vi "Init Condition.vi"(5 "Sequencing":refnum<class "MessageQ.lvclass">, 6 "Variables":refnum<class "Variables.lvclass">, 7 "VolatusAPI":refnum<class "VolatusAPI.lvclass">, 8 "error in (no error)":refnum<class "MultiErrors.lvclass">, 10 "Condition Config":refnum<class "Condition Config.lvclass">, 11 "SeqRunning Condition in":refnum<class "SeqRunning Condition.lvclass">) -> (0 "error out":refnum<class "MultiErrors.lvclass">, 3 "SeqRunning Condition out":refnum<class "SeqRunning Condition.lvclass">)   [LabVIEW 2020, in "VolatusSeq.lvlib" / "SeqRunning Condition.lvclass"]
uses:
  SeqRunning Condition.lvclass
  VolatusErrorUtilities/MultiErrors/MultiErrors.lvclass
  Volatus/VolatusAPI/VolatusAPI.lvclass
  VolatusSeqConfig/Condition Config/Condition Config.lvclass
  Volatus/MessageQ/MessageQ.lvclass
  VolatusSeqConfig/SeqRunning Condition Config/SeqRunning Condition Config.lvclass
  SeqRunning Condition.lvclass/SeqRunning Condition.ctl
  Variables/Variables.lvclass
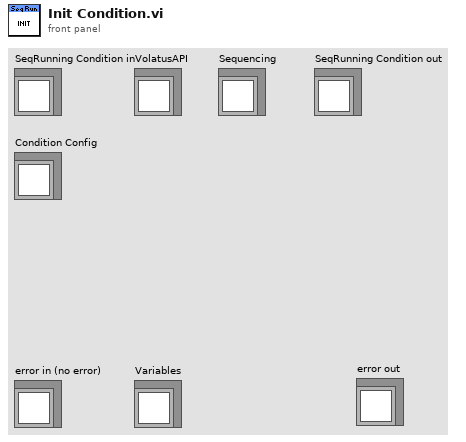
[diagram p1: front panel]
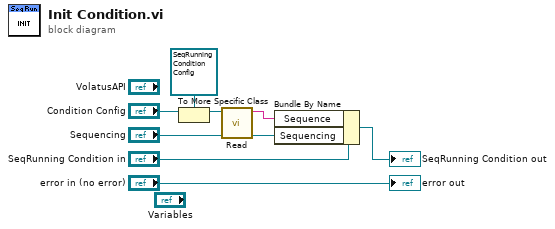
[diagram p0: block diagram]
diagram:
  n1 = To More Specific Class(target class=refnum<class "SeqRunning Condition Config.lvclass"> refnum ("VolatusSeqConfig.lvlib:SeqRunning Condition Config.lvclass"), reference="Condition Config") -> (specific class reference=w5:refnum<class "SeqRunning Condition Config.lvclass">)  [unwired: 1 in, 1 out]
  n2 = call "Read.vi"("SeqRunning Condition Config in"=w5) -> ("Sequence"=w1:string)  [unwired: 10 in]
  n3 = Bundle By Name(cluster="SeqRunning Condition in", "Sequence"=w1, "Sequencing"="Sequencing") -> (→"SeqRunning Condition out":refnum<class "SeqRunning Condition.lvclass">)
  "error out" <- "error in (no error)"
